vi "Update Interface indicator.vi"(8 "error in (no error)":errorcluster, 10 "Interval":dbl, 11 "SPARC4_AC in":refnum<class "S4ACS_GUI.lvclass">) -> (0 "error out":errorcluster, 2 "update indicator?":bool, 3 "SPARC4_AC out":refnum<class "S4ACS_GUI.lvclass">)   [LabVIEW 2018, in "S4ACS_GUI.lvclass"]
uses:
  S4ACS_GUI.lvclass
  S4ACS_GUI.lvclass/S4ACS_GUI.ctl
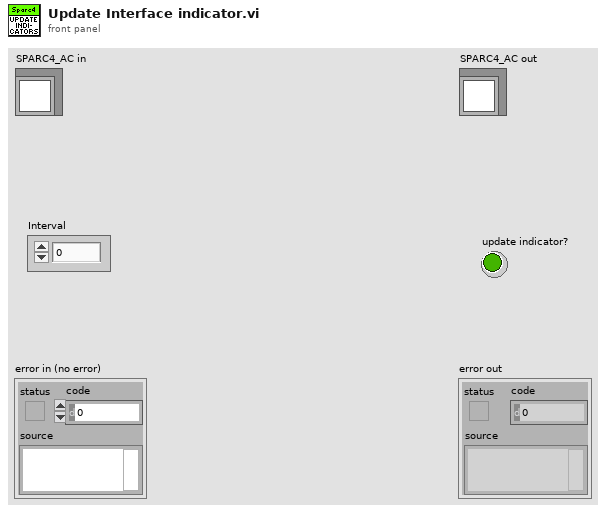
[diagram p1: front panel]
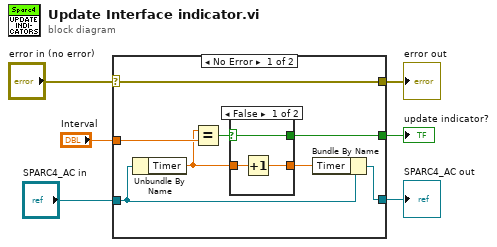
[diagram p0: block diagram]
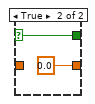
[diagram p2: hidden frame]
diagram:
  n1 = case shown="No Error" "error in (no error)" {
    selector: "error in (no error)" -> [w14 w21]
    tunnel: [w14 w21] -> w5
    tunnel: [w9 w20] -> w3
    tunnel: "SPARC4_AC in" -> [w10 w20]
    tunnel: "Interval" -> [w13 _]
    tunnel: [w11 _] -> w1
    frame No Error {
      n2 = Unbundle By Name(w10) -> ("Timer"=w7:dbl)
      n3 = Equal?(x=w7, y=w13) -> (x = y?=w12:bool)
      n4 = case shown="False" w12 {
        selector: w12 -> [w15 w19]
        tunnel: [w15 w19] -> w11
        tunnel: [w16 0.0] -> w8
        tunnel: w7 -> [w17 _]
        frame False {
          n5 = Increment(x=w17) -> (x+1=w16:dbl)
        }
        frame True {
        }
      }
      n6 = Bundle By Name(cluster=w10, "Timer"=w8) -> (w9:refnum<class "S4ACS_GUI.lvclass">)
    }
    frame Error {
    }
  }
  "error out" <- w5
  "SPARC4_AC out" <- w3
  "update indicator?" <- w1
